vi "GenericIMAQGetConfig.vi"(10 "Camera (in)":T1={"Framerate (Hz)"=100, "Exposure time (us)"=100, "Image size"={"Width"=1280, "Height"=1024}, "Number of buffers"=30}, 11 "IMAQ Refnum in":refnum<k11>) -> (2 "Camera":T1={"Framerate (Hz)"=100, "Exposure time (us)"=100, "Image size"={"Width"=1280, "Height"=1024}, "Number of buffers"=30}, 3 "IMAQ Session Out":refnum<k11>)   [LabVIEW 2011]
uses:
  Main/Camera/GenericCameraConfigType.ctl
  Global_GenericIMAQCamera_HardwareConfig.vi
panel:
  out "framerate":i32
  out "Exposure Time (us)":i32
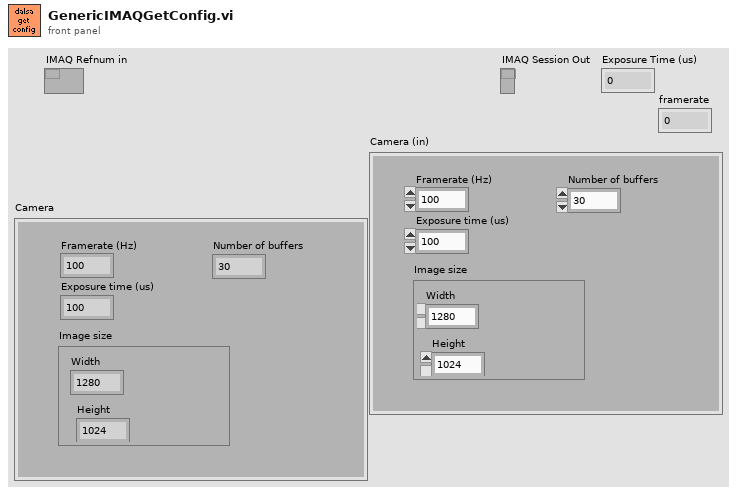
[diagram p1: front panel]
types:
  T1 = typedef "GenericCameraConfigType.ctl" = cluster{"Framerate (Hz)":i32, "Exposure time (us)":i32, "Image size":cluster{"Width":i32, "Height":i32}, "Number of buffers":i32}
  T2 = typedef "GenericIMAQHardwareConfig.ctl" = cluster{"Use serial commands directly":bool, "Frame rate set cmd":string, "Exposure time set cmd":string, "Frame rate get cmd":string, "Exposure time get cmd":string, "IMAQ Identifier":string, "Serial return skip chars":i32, "Set width/height":string, "Set offset xy":string, "Get width":string, "Get height":string, "Get offset X":string, "Get offset Y":string, "Full frame size":cluster{"width":i32, "height":i32}}
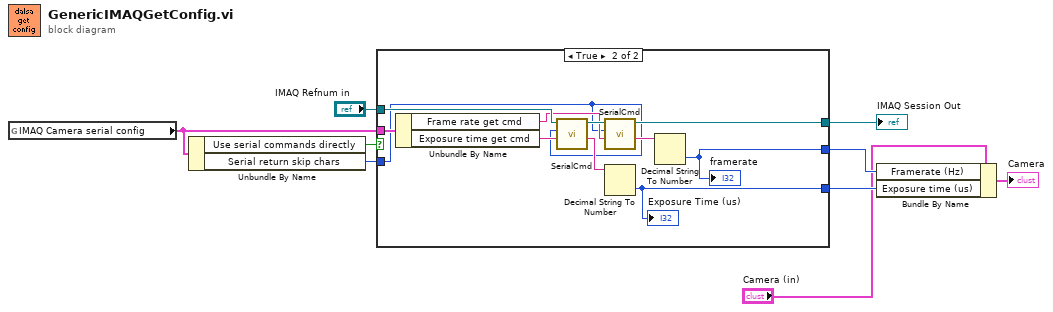
[diagram p0: block diagram]
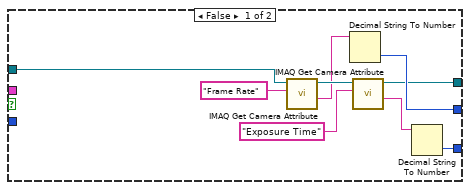
[diagram p2: hidden frame]
diagram:
  n1 = global read "Global_GenericIMAQCamera_HardwareConfig.vi" "IMAQ Camera serial config"() -> (w2:T2)
  n2 = Unbundle By Name(w2) -> ("Use serial commands directly"=w3:bool, "Serial return skip chars"=w1:i32)
  n3 = case shown="True" w3 {
    tunnel: "IMAQ Refnum in" -> [w10 w29]
    tunnel: [w12 w28] -> w8
    tunnel: [w14 w27] -> w7
    tunnel: [w11 w23] -> w4
    tunnel: w2 -> [_ w22]
    tunnel: w1 -> [_ w19]
    frame False {
      n4 = call <vilib>:"IMAQ Get Camera Attribute.vi"("Camera Attribute"="Frame Rate", "IMAQ Session In"=w10) -> ("Attribute Value"=w13:string, "IMAQ Session Out"=w18:refnum<k11>)  [unwired: 5 in, 1 out]
      n5 = Decimal String To Number(string=w13) -> (number=w12:i32)  [unwired: 2 in, 1 out]
      n6 = call <vilib>:"IMAQ Get Camera Attribute.vi"("Camera Attribute"="Exposure Time", "IMAQ Session In"=w18) -> ("Attribute Value"=w15:string, "IMAQ Session Out"=w11:refnum<k11>)  [unwired: 5 in, 1 out]
      n7 = Decimal String To Number(string=w15) -> (number=w14:i32)  [unwired: 2 in, 1 out]
    }
    frame True {
      n8 = Unbundle By Name(w22) -> ("Frame rate get cmd"=w20:string, "Exposure time get cmd"=w21:string)
      n9 = call "SerialCmd.vi"("command"=w21, "Return string skip chars (2)"=w19, "IMAQ Refnum in"=w29) -> ("String Read"=w25:string, "IMAQ Session Out"=w26:refnum<k11>)  [unwired: 5 in, 2 out]
      n10 = call "SerialCmd.vi"("command"=w20, "Return string skip chars (2)"=w19, "IMAQ Refnum in"=w26) -> ("String Read"=w24:string, "IMAQ Session Out"=w23:refnum<k11>)  [unwired: 5 in, 2 out]
      n11 = Decimal String To Number(string=w25) -> (number=w27:i32)  [unwired: 2 in, 1 out]
      "Exposure Time (us)" <- w27
      n12 = Decimal String To Number(string=w24) -> (number=w28:i32)  [unwired: 2 in, 1 out]
      "framerate" <- w28
    }
  }
  "IMAQ Session Out" <- w4
  n13 = Bundle By Name(cluster="Camera (in)", "Framerate (Hz)"=w8, "Exposure time (us)"=w7) -> (→"Camera":T1)
